vi "1.4nad.vi"() -> ()   [LabVIEW 2020]
uses:
  <vilib>/measure/NI_MABase.lvlib
panel:
  in  "Cluster":cluster{"Sampling Freq":dbl, "Samples":dbl}
  in  "Signal type":u16(ring) items=["Sine Wave", "Triangle Wave", "Square Wave", "Sawtooth Wave"]
  in  "Signal class":u16(ring) items=["Noise", "Periodic"]
  in  "Czestotliwosc":dbl(knob) scale=0.01..500.0
  in  "Amplituda":dbl(knob) scale=0.01..10.0
  in  "stop":bool
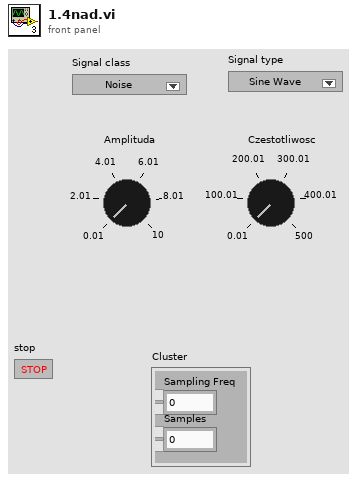
[diagram p1: front panel]
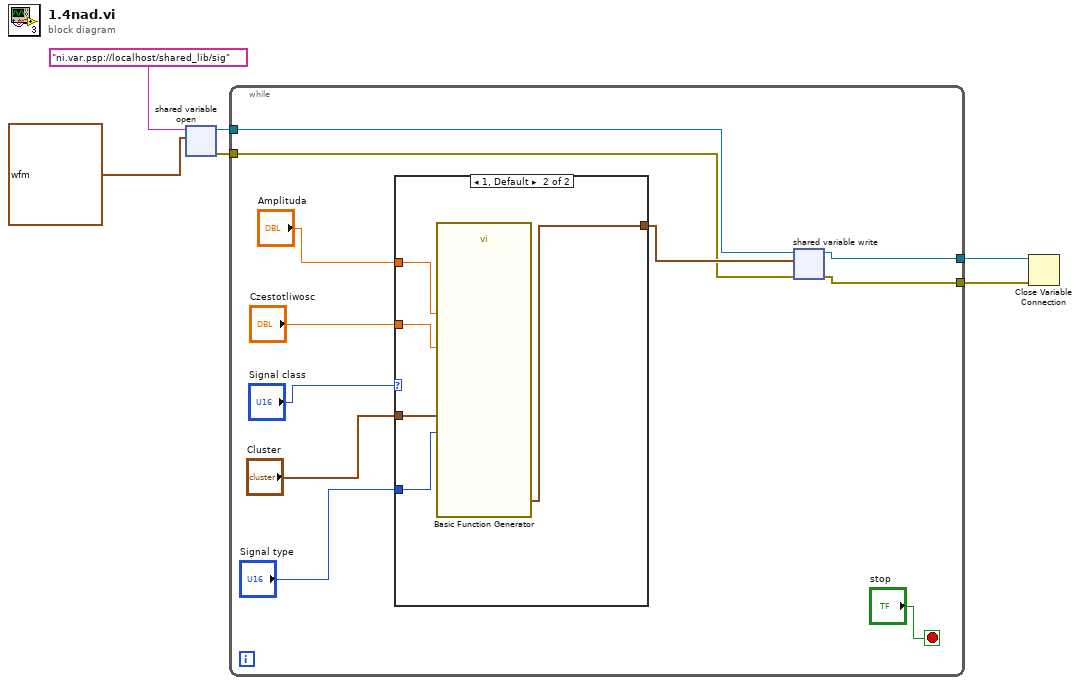
[diagram p0: block diagram]
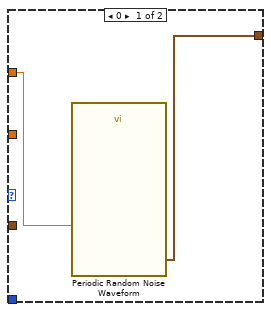
[diagram p2: hidden frame]
diagram:
  n1 = shared-variable-open("ni.var.psp://localhost/shared_lib/sig", waveform(dbl) {"t0"=timestamp(0 s since 1904-01-01), "dt"=1.0, "Y"=[]} ("Waveform")) -> (w5:refnum<k21>, w2:errorcluster)  [unwired: 2 in]
  n2 = while {
    tunnel: w5 -> [w11]
    tunnel: [w9] -> w4
    tunnel: [w8] -> w3
    tunnel: w2 -> [w7]
    stop <- "stop" stop-if-true
    n3 = case shown="1, Default" "Signal class" {
      tunnel: "Amplituda" -> [w19 w24]
      tunnel: "Czestotliwosc" -> [_ w23]
      tunnel: "Signal type" -> [_ w22]
      tunnel: [w18 w21] -> w10
      tunnel: "Cluster" -> [_ w20]
      frame 0 {
        n4 = call <vilib>:"Periodic Random Noise Waveform.vi"("spectral amplitude"=w19) -> ("signal out"=w18:waveform(dbl))  [unwired: 9 in, 1 out]
      }
      frame 1, Default {
        n5 = call <vilib>:"Basic Function Generator.vi"("sampling info"=w20, "signal type"=w22, "amplitude"=w24, "frequency"=w23) -> ("signal out"=w21:waveform(dbl))  [unwired: 5 in, 2 out]
      }
    }
    n6 = shared-variable-write(w11, w7, w10) -> (w8:refnum<k21>, w9:errorcluster)
  }
  n7 = Close Variable Connection(8:w4, 11:w3) -> ()  [unwired: 1 out]
